vi "metadata grab based on inst ctrl states.vi"(0 "ComboBox in":refnum<vi>, 1 "sphere":refnum<vi>, 2 "Instrument Control \nSwitches":T3, 5 "Analyzer Choice":T2, 7 "spectrometer":refnum<vi>, 9 "ampGainRange":refnum<vi>, 11 "error in (no error)":errorcluster, 12 "Sphere Indicator":T1=enum."Insulated Sphere", 13 "analyzer":refnum<vi>) -> (15 "error out":errorcluster)   [LabVIEW 2013]
uses:
  Instrument Control Switches.ctl
  Analyzer Choice.ctl
  avantesSpectrometer/Acquisition/Sphere Indicator.ctl
  avantesSpectrometer/AvaSpec.lvlib
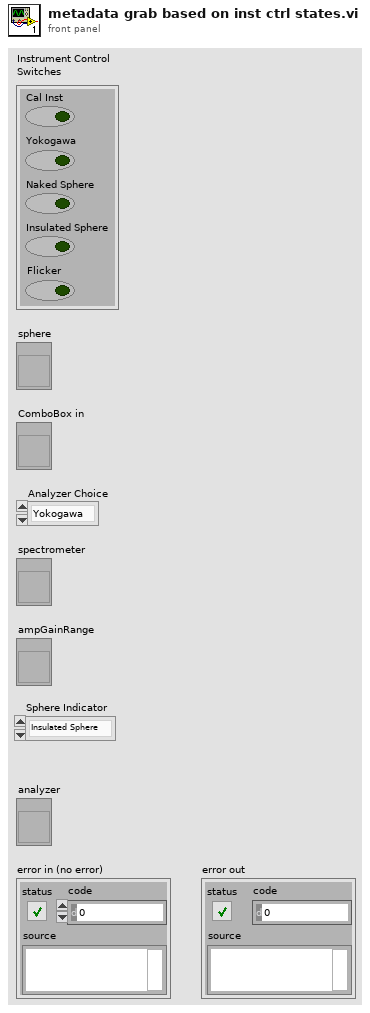
[diagram p1: front panel]
types:
  T1 = typedef "AvaSpec.lvlib/Sphere Indicator.ctl" = enum16{"Naked Sphere", "Insulated Sphere"}
  T2 = typedef "Analyzer Choice.ctl" = enum16{"Yokogawa", "Cal Inst"}
  T3 = typedef "Instrument Control Switches.ctl" = cluster{"Cal Inst":bool, "Yokogawa":bool, "Naked Sphere":bool, "Insulated Sphere":bool, "Flicker":bool}
  T4 = enum8{"Enabled", "Disabled", "Disabled and Grayed Out"}
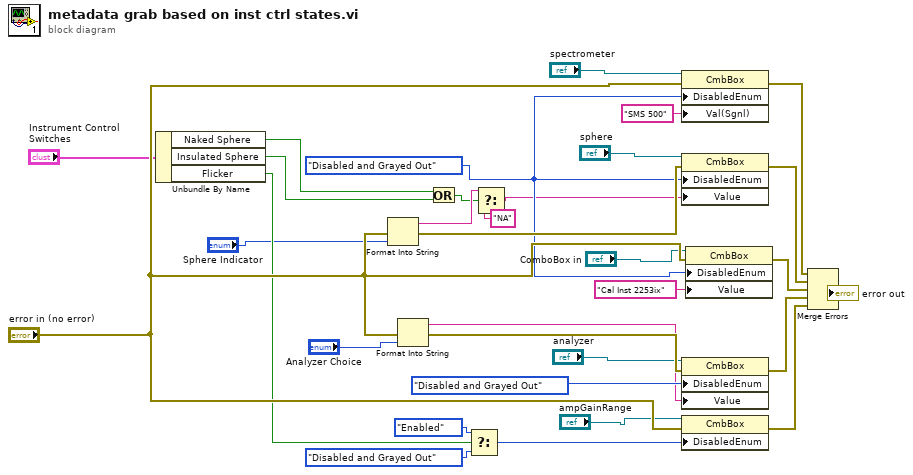
[diagram p0: block diagram]
diagram:
  w17 = T4."Disabled and Grayed Out" ("Disabled")
  n1 = Unbundle By Name("Instrument Control \nSwitches") -> ("Naked Sphere"=w10:bool, "Insulated Sphere"=w11:bool, "Flicker"=w6:bool)
  n2 = Format Into String(error in="error in (no error)", "Sphere Indicator") -> (resulting string=w13:string, error out=w24:errorcluster)  [unwired: 2 in]
  n3 = Format Into String(error in="error in (no error)", "Analyzer Choice") -> (resulting string=w9:string, error out=w25:errorcluster)  [unwired: 2 in]
  n4 = Or(x=w10, y=w11) -> (x .or. y?=w12:bool)
  n5 = Select(t=T4."Enabled" ("Disabled"), s=w6, f=T4."Disabled and Grayed Out" ("Disabled")) -> (s? t:f=w5:T4)
  n6 = Select(t=w13, s=w12, f="NA") -> (s? t:f=w14:string)
  n7 = property class="CmbBox"(reference="spectrometer", error in="error in (no error)", "DisabledEnum"=w17, "Val(Sgnl)"="SMS 500" ("Value")) -> (error out=w29:errorcluster)  [unwired: 1 out]
  n8 = property class="CmbBox"(reference="sphere", error in=w24, "DisabledEnum"=w17, "Value"=w14) -> (error out=w28:errorcluster)  [unwired: 1 out]
  n9 = property class="CmbBox"(reference="analyzer", error in=w25, "DisabledEnum"=T4."Disabled and Grayed Out" ("Disabled"), "Value"=w9) -> (error out=w30:errorcluster)  [unwired: 1 out]
  n10 = property class="CmbBox"(reference="ampGainRange", error in="error in (no error)", "DisabledEnum"=w5) -> (error out=w31:errorcluster)  [unwired: 1 out]
  n11 = property class="CmbBox"(reference="ComboBox in", error in="error in (no error)", "DisabledEnum"=w17, "Value"="Cal Inst 2253ix") -> (error out=w27:errorcluster)  [unwired: 1 out]
  n12 = Merge Errors(w29, w28, w27, w30, w31) -> (→"error out":errorcluster)
